vi "provide_OME_data.vi"(6 "image ID":string, 8 "error in (no error)":errorcluster, 9 "structuredAttribute string in":string, 10 "OME element in":refnum<class "XMLElement.lvclass">, 11 "GenericObjective in":refnum<class "GenericObjective.lvclass">) -> (0 "error out":errorcluster, 1 "structuredAttribute string out":string, 2 "OME element out":refnum<class "XMLElement.lvclass">, 3 "GenericObjective out":refnum<class "GenericObjective.lvclass">)   [LabVIEW 2010, in "GenericObjective.lvclass"]
uses:
  GenericObjective.lvclass
  common/classes/XMLElement/XMLElement/XMLElement.lvclass
  common/classes/GenericComponent/GenericComponent/GenericComponent.lvclass
  Instrument/GenericInstrument/GenericInstrument/GenericInstrument.lvclass
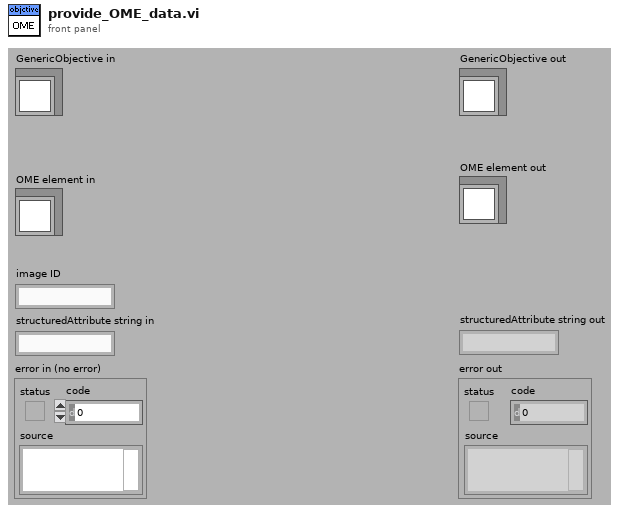
[diagram p1: front panel]
types:
  T1 = typedef "GenericObjective.lvclass/correction_enum.ctl" = enum16{"UV", "PlanApo", "PlanFluor", "SuperFluor", "VioletCorrected", "Unknown"}
  T2 = typedef "GenericObjective.lvclass/immersion_enum.ctl" = enum16{"Oil", "Water", "WaterDipping", "Air", "Multi", "Glycerol", "Other", "Unknown"}
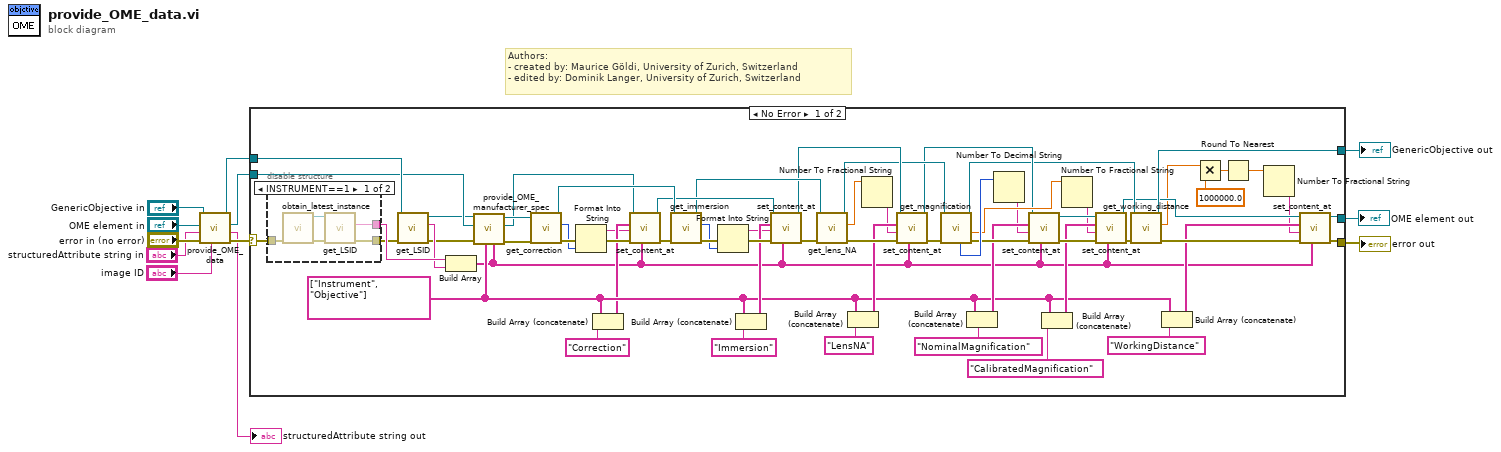
[diagram p0: block diagram]
diagram:
  # "Authors: \n- created by: Maurice Göldi, University of Zurich, Switzerland\n- edited by: Dominik Langer, University of Zurich, Switzerland"
  n1 = call-parent "provide_OME_data.vi"("image ID"="image ID", "error in (no error)"="error in (no error)", "structuredAttribute string in"="structuredAttribute string in", "OME element in"="OME element in", "GenericPlugin in"="GenericObjective in") -> ("error out"=w8:errorcluster, "structuredAttribute string out"=→"structuredAttribute string out":string, "OME element out"=w6:refnum<class "XMLElement.lvclass">, "GenericPlugin out"=w7:refnum<class "GenericObjective.lvclass">)  [unwired: 3 in]
  n2 = case shown="No Error" w8 {
    selector: w8 -> [w76 w85]
    tunnel: [w72 w85] -> w12
    tunnel: [w73 w84] -> w11
    tunnel: w7 -> [w75 w84]
    tunnel: w6 -> [w74 w83]
    tunnel: [w71 w83] -> w4
    frame No Error {
      w21 = string[] ["Instrument", "Objective"]
      n3 = disable-structure shown="INSTRUMENT==1" {
        disable-tunnel: w76 -> [w79 w82]
        disable-tunnel: [w78 w82] -> w62
        disable-tunnel: [w77 _] -> w63
        frame condition #0 {
          n4 = call "obtain_latest_instance.vi"("error in (no error)"=w79) -> ("error out"=w80:errorcluster, "microscope"=w81:refnum<class "GenericInstrument.lvclass">)  [unwired: 9 in]
          n5 = call-dynamic "get_LSID.vi"("error in (no error)"=w80, "GenericPlugin in"=w81) -> ("error out"=w78:errorcluster, "LSID (string)"=w77:string)  [unwired: 6 in, 2 out]
        }
        frame condition #1 (active) {
        }
      }
      n6 = call-dynamic "get_LSID.vi"("error in (no error)"=w62, "GenericPlugin in"=w75) -> ("error out"=w60:errorcluster, "LSID (string)"=w61:string, "GenericPlugin out"=w59:refnum<class "GenericObjective.lvclass">)  [unwired: 6 in, 1 out]
      n7 = Build Array(w63, w61) -> (w19:string[])
      n8 = call-dynamic "provide_OME_manufacturer_spec.vi"("id chain"=w19, "key chain"=w21, "error in (no error)"=w60, "XMLElement in"=w74, "GenericPlugin in"=w59) -> ("error out"=w58:errorcluster, "XMLElement out"=w54:refnum<class "XMLElement.lvclass">, "GenericPlugin out"=w57:refnum<class "GenericObjective.lvclass">)  [unwired: 4 in]
      n9 = call-dynamic "get_correction.vi"("error in (no error)"=w58, "GenericObjective in"=w57) -> ("error out"=w67:errorcluster, "Correction"=w66:T1, "GenericObjective out"=w70:refnum<class "GenericObjective.lvclass">)  [unwired: 7 in]
      n10 = Format Into String(error in=w67, w66) -> (resulting string=w17:string, error out=w56:errorcluster)  [unwired: 2 in]
      n11 = Build Array (concatenate)(w21, "Correction") -> (w20:string[])
      n12 = call "set_content_at.vi"("id chain"=w19, "error in (no error)"=w56, "content"=w17, "key chain"=w20, "Element in"=w54) -> ("error out"=w55:errorcluster, "Element out"=w52:refnum<class "XMLElement.lvclass">)  [unwired: 5 in]
      n13 = call-dynamic "get_immersion.vi"("error in (no error)"=w55, "GenericObjective in"=w70) -> ("error out"=w65:errorcluster, "Immersion"=w64:T2, "GenericObjective out"=w49:refnum<class "GenericObjective.lvclass">)  [unwired: 7 in]
      n14 = Format Into String(error in=w65, w64) -> (resulting string=w16:string, error out=w53:errorcluster)  [unwired: 2 in]
      n15 = Build Array (concatenate)(w21, "Immersion") -> (w51:string[])
      n16 = call "set_content_at.vi"("id chain"=w19, "error in (no error)"=w53, "content"=w16, "key chain"=w51, "Element in"=w52) -> ("error out"=w50:errorcluster, "Element out"=w43:refnum<class "XMLElement.lvclass">)  [unwired: 5 in]
      n17 = call-dynamic "get_lens_NA.vi"("error in (no error)"=w50, "GenericObjective in"=w49) -> ("error out"=w47:errorcluster, "lens NA"=w48:dbl, "GenericObjective out"=w40:refnum<class "GenericObjective.lvclass">)  [unwired: 7 in]
      n18 = Build Array (concatenate)(w21, "LensNA") -> (w45:string[])
      n19 = Number To Fractional String(number=w48) -> (F-format string=w15:string)  [unwired: 3 in]
      n20 = call "set_content_at.vi"("id chain"=w19, "error in (no error)"=w47, "content"=w15, "key chain"=w45, "Element in"=w43) -> ("error out"=w44:errorcluster, "Element out"=w35:refnum<class "XMLElement.lvclass">)  [unwired: 5 in]
      n21 = call-dynamic "get_magnification.vi"("error in (no error)"=w44, "GenericObjective in"=w40) -> ("error out"=w41:errorcluster, "calibrated magnification"=w37:dbl, "GenericObjective out"=w32:refnum<class "GenericObjective.lvclass">, "nominal magnification"=w42:i32)  [unwired: 5 in, 1 out]
      n22 = Build Array (concatenate)(w21, "NominalMagnification") -> (w38:string[])
      n23 = Number To Decimal String(number=w42) -> (decimal integer string=w14:string)  [unwired: 1 in]
      n24 = call "set_content_at.vi"("id chain"=w19, "error in (no error)"=w41, "content"=w14, "key chain"=w38, "Element in"=w35) -> ("error out"=w34:errorcluster, "Element out"=w36:refnum<class "XMLElement.lvclass">)  [unwired: 5 in]
      n25 = Build Array (concatenate)(w21, "CalibratedMagnification") -> (w27:string[])
      n26 = Number To Fractional String(number=w37) -> (F-format string=w13:string)  [unwired: 3 in]
      n27 = call "set_content_at.vi"("id chain"=w19, "error in (no error)"=w34, "content"=w13, "key chain"=w27, "Element in"=w36) -> ("error out"=w33:errorcluster, "Element out"=w30:refnum<class "XMLElement.lvclass">)  [unwired: 5 in]
      n28 = call-dynamic "get_working_distance.vi"("error in (no error)"=w33, "GenericObjective in"=w32) -> ("error out"=w31:errorcluster, "working distance"=w24:dbl[unit], "GenericObjective out"=w73:refnum<class "GenericObjective.lvclass">)  [unwired: 7 in]
      n29 = Build Array (concatenate)(w21, "WorkingDistance") -> (w26:string[])
      n30 = Multiply(x=w24, y=dbl[unit] 1000000.0) -> (x*y=w25:dbl)
      n31 = Round To Nearest(number=w25) -> (nearest integer value=w22:dbl)
      n32 = Number To Fractional String(number=w22) -> (F-format string=w18:string)  [unwired: 3 in]
      n33 = call "set_content_at.vi"("id chain"=w19, "error in (no error)"=w31, "content"=w18, "key chain"=w26, "Element in"=w30) -> ("error out"=w72:errorcluster, "Element out"=w71:refnum<class "XMLElement.lvclass">)  [unwired: 5 in]
    }
    frame Error {
    }
  }
  "error out" <- w12
  "GenericObjective out" <- w11
  "OME element out" <- w4
